vi "布尔数组处理.vi"(10 "数组":bool[](array[boolean])) -> (0 "元素 6":bool, 1 "元素 5":bool, 2 "元素 4":bool, 3 "元素 3":bool, 4 "元素 7":bool, 5 "元素 2":bool, 6 "元素 8":bool, 7 "元素":bool)   [LabVIEW 2018]
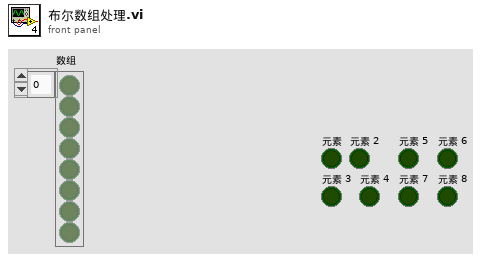
[diagram p1: front panel]
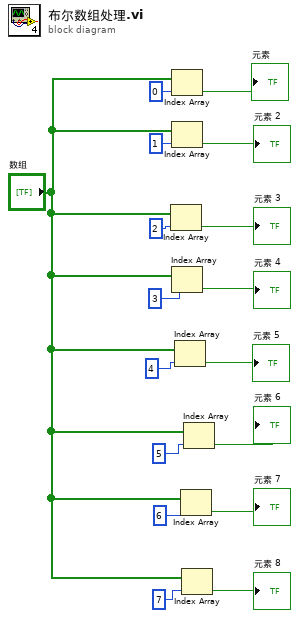
[diagram p0: block diagram]
diagram:
  n1 = Index Array(array="数组", index=2 ("索引")) -> (element=→"元素 3":bool)
  n2 = Index Array(array="数组", index=0 ("索引")) -> (element=→"元素":bool)
  n3 = Index Array(array="数组", index=1 ("索引")) -> (element=→"元素 2":bool)
  n4 = Index Array(array="数组", index=3 ("索引")) -> (element=→"元素 4":bool)
  n5 = Index Array(array="数组", index=4 ("索引")) -> (element=→"元素 5":bool)
  n6 = Index Array(array="数组", index=6 ("索引")) -> (element=→"元素 7":bool)
  n7 = Index Array(array="数组", index=7 ("索引")) -> (element=→"元素 8":bool)
  n8 = Index Array(array="数组", index=5 ("索引")) -> (element=→"元素 6":bool)
